vi "delete channel from configuration.vi"(8 "error in":errorcluster, 10 "Modbus Module Channel.lvclass":refnum<class "Modbus Module Channel.lvclass">, 11 "Modbus Slave configuration in":refnum<class "Modbus Slave configuration.lvclass">) -> (0 "error out":errorcluster, 3 "Modbus Slave configuration out":refnum<class "Modbus Slave configuration.lvclass">)   [LabVIEW 2013, in "Modbus Slave configuration.lvclass"]
doc: "Platypus Framework 1.0.1.65\nNI Systems Engineering - National Instruments"
uses:
  Modbus Slave configuration.lvclass
  module channel/Modbus Module Channel.lvclass
  <vilib>/NI/Tag Bus/tag/tag descriptor.lvclass/tag descriptor.ctl
  Modbus Slave configuration.lvclass/Modbus Slave configuration.ctl
  <vilib>/NI/Tag Bus/tag/tag descriptor.lvclass
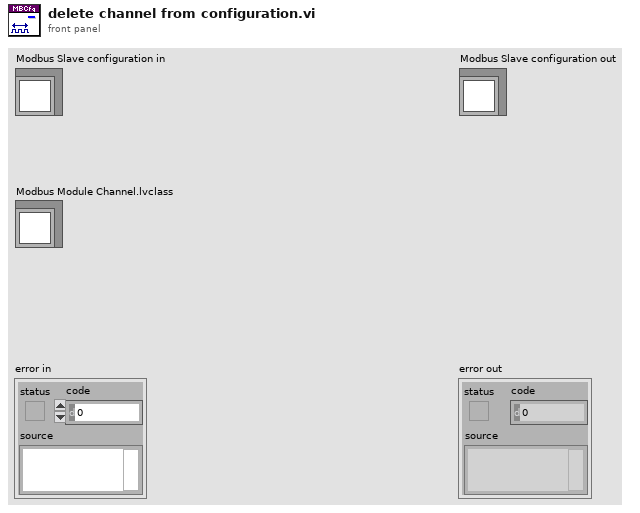
[diagram p1: front panel]
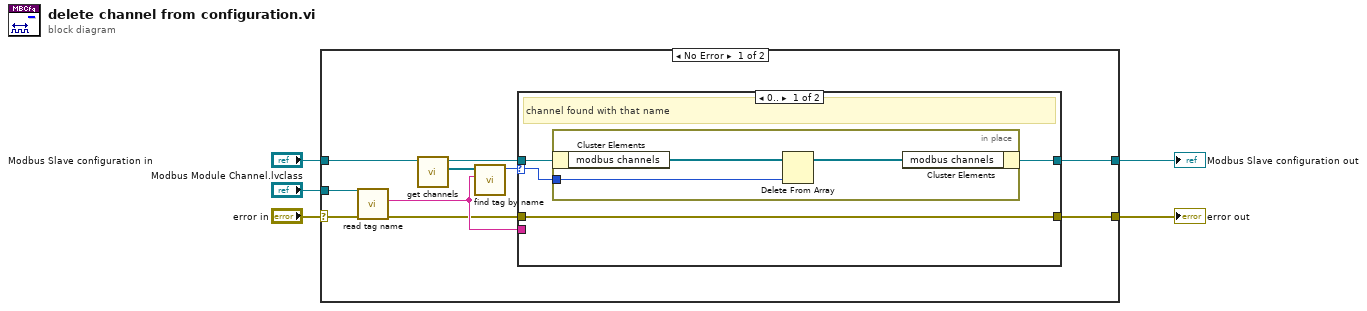
[diagram p0: block diagram]
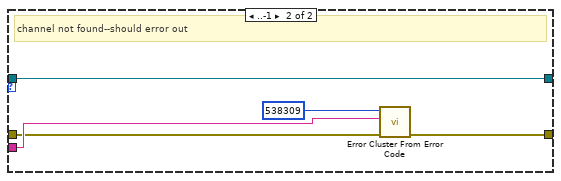
[diagram p2: hidden frame]
diagram:
  n1 = case shown="No Error" "error in" {
    selector: "error in" -> [w8 w28]
    tunnel: "Modbus Module Channel.lvclass" -> [w14 _]
    tunnel: [w13 w28] -> w4
    tunnel: [w12 w29] -> w3
    tunnel: "Modbus Slave configuration in" -> [w11 w29]
    frame No Error {
      n2 = call <vilib>:"read tag name.vi"("error in"=w8, "system tag in"=w14) -> ("error out"=w6:errorcluster, "name"=w7:string)  [unwired: 7 in, 1 out]
      n3 = call-dynamic "get channels.vi"("Modbus Slave configuration in"=w11) -> ("channels"=w10:refnum<class "TBM channel.lvclass">[], "Modbus Slave configuration out"=w15:refnum<class "Modbus Slave configuration.lvclass">)  [unwired: 9 in]
      n4 = call <vilib>:"find tag by name.vi"("name"=w7, "tags in"=w10) -> ("index"=w9:i32)  [unwired: 9 in]
      n5 = case shown="0.." w9 {
        selector: w9 -> [w19 _]
        tunnel: [w16 w27] -> w13
        tunnel: w7 -> [_ w25]
        tunnel: w6 -> [w16 w24]
        tunnel: w15 -> [w18 w23]
        tunnel: [w17 w23] -> w12
        frame 0.. {
          # "channel found with that name"
          n6 = in-place {
            in-place-border: w19 -> [w22]
            n7 = in-place-cluster #1(w18) -> ("modbus channels"=w21:refnum<class "Modbus Module Channel.lvclass">[])
            n8 = Delete From Array(array=w21, index=w22) -> (array with subset deleted=w20:refnum<class "Modbus Module Channel.lvclass">[])  [unwired: 1 in, 1 out]
            n9 = in-place-cluster #1("modbus channels"=w20) -> (w17:refnum<class "Modbus Slave configuration.lvclass">)
          }
        }
        frame ..-1 {
          # "channel not found--should error out"
          n10 = call <vilib>:"Error Cluster From Error Code.vi"("error in (no error)"=w24, "error message (\"\")"=w25, "error code (0)"=538309) -> ("error out"=w27:errorcluster)  [unwired: 6 in]
        }
      }
    }
    frame Error {
    }
  }
  "error out" <- w4
  "Modbus Slave configuration out" <- w3
